vi "CI-recieveStatus.vi"(8 "error in (no error)":errorcluster, 10 "status":T1, 11 "common-interface in":refnum<class "VDH-VNA_data_handler.lvclass">) -> (0 "error out":errorcluster, 3 "common-interface out":refnum<class "VDH-VNA_data_handler.lvclass">)   [LabVIEW 2020, in "VDH-VNA_data_handler.lvlib" / "VDH-VNA_data_handler.lvclass"]
uses:
  VDH-VNA_data_handler.lvclass
  common/interface/CI-common_interface/CI-status_clust.ctl
  common/interface/CI-common_interface/CI-module_enum.ctl
  common/interface/CI-common_interface/CI-common_interface.lvclass
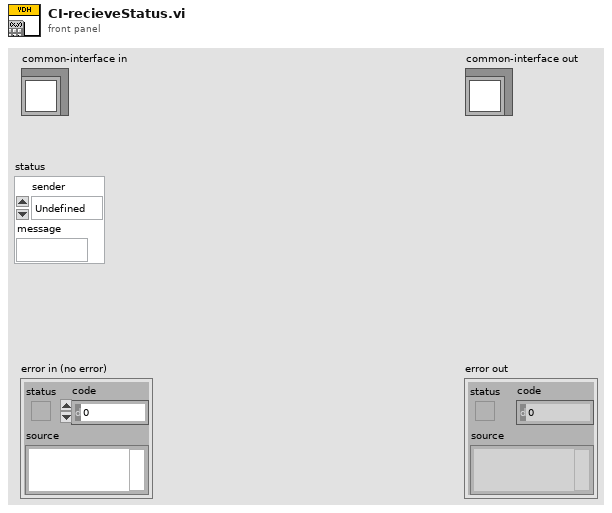
[diagram p1: front panel]
types:
  T1 = typedef "CI-common_interface.lvlib/CI-common_interface.lvclass/CI-status_clust.ctl" = cluster{"sender":T2, "message":string}
  T2 = typedef "CI-common_interface.lvlib/CI-common_interface.lvclass/CI-module_enum.ctl" = enum16{"Undefined", "HWM", "VDH", "GUI"}
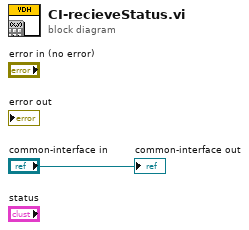
[diagram p0: block diagram]
diagram:
  "common-interface out" <- "common-interface in"
